vi "Parse Sensor Group 5.vi"(11 "stream in":u8[](array[numeric])) -> (1 "Sensor Group 5":T1, 3 "stream out":u8[](array[numeric]))   [LabVIEW 2015]
doc: "Read Sensor Group 5 from a UART data stream."
uses:
  Sensor Group 5.ctl
  OI Mode.ctl
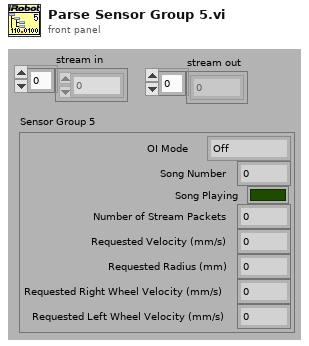
[diagram p1: front panel]
types:
  T1 = typedef "Sensor Group 5.ctl" = cluster{"OI Mode":T2, "Song Number":u8, "Song Playing":bool, "Number of Stream Packets":u8, "Requested Velocity (mm/s)":i16, "Requested Radius (mm)":i16, "Requested Right Wheel Velocity (mm/s)":i16, "Requested Left Wheel Velocity (mm/s)":i16}
  T2 = typedef "OI Mode.ctl" = enum16{"Off", "Passive", "Safe", "Full"}
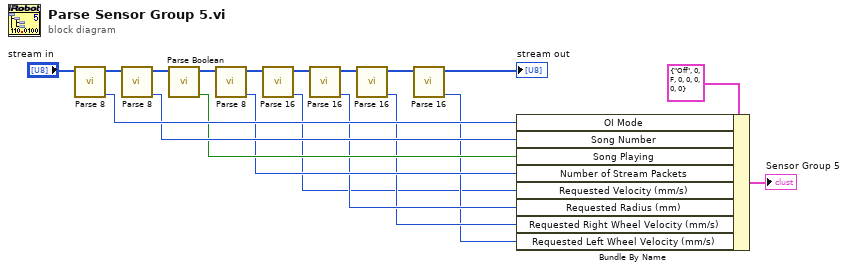
[diagram p0: block diagram]
diagram:
  n1 = call "Parse 8.vi"("stream in"="stream in") -> ("value"=w16:u8, "stream out"=w15:u8[])  [unwired: 9 out]
  n2 = call "Parse 8.vi"("stream in"=w15) -> ("value"=w14:u8, "stream out"=w13:u8[])  [unwired: 9 out]
  n3 = call "Parse Boolean.vi"("stream in"=w13) -> ("Value"=w12:bool, "stream out"=w11:u8[])  [unwired: 9 out]
  n4 = call "Parse 8.vi"("stream in"=w11) -> ("value"=w10:u8, "stream out"=w9:u8[])  [unwired: 9 out]
  n5 = call "Parse 16.vi"("stream in"=w9) -> ("value"=w1:u16, "stream out"=w8:u8[])  [unwired: 9 out]
  n6 = call "Parse 16.vi"("stream in"=w8) -> ("value"=w7:u16, "stream out"=w6:u8[])  [unwired: 9 out]
  n7 = call "Parse 16.vi"("stream in"=w6) -> ("value"=w5:u16, "stream out"=w4:u8[])  [unwired: 9 out]
  n8 = call "Parse 16.vi"("stream in"=w4) -> ("value"=w3:u16, "stream out"=→"stream out":u8[])  [unwired: 9 out]
  n9 = Bundle By Name(cluster=T1 {"OI Mode"=enum."Off", "Song Number"=0, "Song Playing"=FALSE, "Number of Stream Packets"=0, "Requested Velocity (mm/s)"=0, "Requested Radius (mm)"=0, "Requested Right Wheel Velocity (mm/s)"=0, "Requested Left Wheel Velocity (mm/s)"=0} ("Sensor Group 5"), "OI Mode"=w16, "Song Number"=w14, "Song Playing"=w12, "Number of Stream Packets"=w10, "Requested Velocity (mm/s)"=w1, "Requested Radius (mm)"=w7, "Requested Right Wheel Velocity (mm/s)"=w5, "Requested Left Wheel Velocity (mm/s)"=w3) -> (→"Sensor Group 5":T1)
